vi "Untitled 1.vi"() -> ()   [LabVIEW 2017]
uses:
  <userlib>/_OpenG.lib/array/array.llb/Remove Duplicates from 1D Array (String)__ogtk.vi
  <userlib>/_OpenG.lib/array/array.llb/Index 1D Array Elements (String)__ogtk.vi
panel:
  out "Duplicates":string[](array[string])
  out "indices of removed elements":i32[](array[numeric])
  out "Array":string[](array[string])
  out "Error (out)":errorcluster
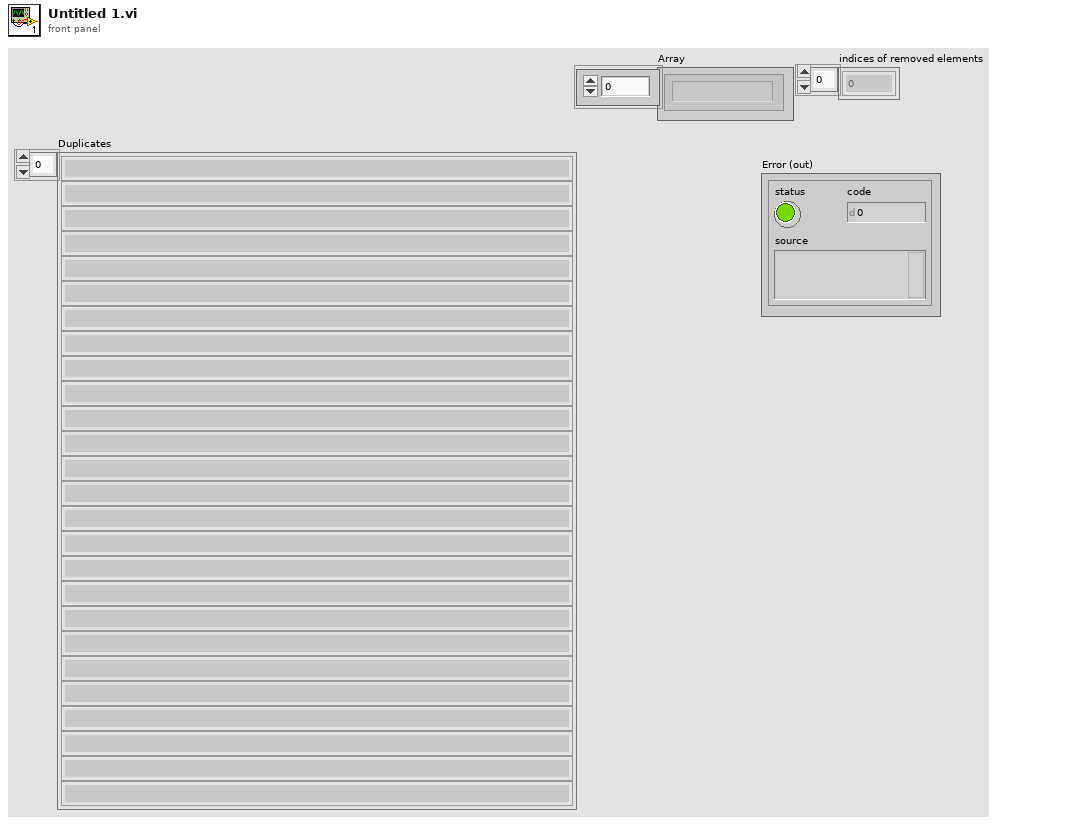
[diagram p1: front panel]
types:
  T1 = typedef "Database_Array.ctl" = cluster{"Core Number":i32, "Channel Number":i32, "Channel Name":string, "Channel Speed":i32, "Label Decimal":i32, "Label Name":string, "Min Rate (mS)":i32, "Max Rate (mS)":i32, "SDI":i32, "SSM":i32, "Create SDI":bool, "Create SSM":bool, "Create Parity":bool, "Parameter Name":string, "Start Bit":i32, "Number of Bits":i32, "Scale":string, "Offset":string, "Signed":bool, "Unit":string, "Encoding":T2, "Default Value":string}
  T2 = typedef "Encoding.ctl" = enum16{"BCD", "BNR", "Discrete"}
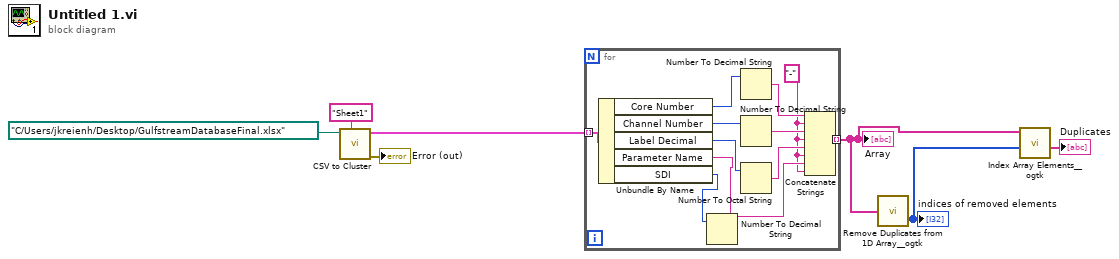
[diagram p0: block diagram]
diagram:
  n1 = call "CSV to Cluster.vi"("Excel._SheetName"="Sheet1", "file path (dialog if empty)"=path "C:/Users/jkreienh/Desktop/GulfstreamDatabaseFinal.xlsx") -> ("Error (out)"=→"Error (out)":errorcluster, "Parameter Array"=w4:T1[])  [unwired: 8 in]
  n2 = for {
    tunnel: w4 -> [w18] mode=indexing
    tunnel: [w11] -> w3 mode=indexing
    w9 = "-"
    n3 = Unbundle By Name(w18) -> ("Core Number"=w17:i32, "Channel Number"=w16:i32, "Label Decimal"=w15:i32, "Parameter Name"=w10:string, "SDI"=w8:i32)
    n4 = Number To Decimal String(number=w8) -> ()  [unwired: 1 in, 1 out]
    n5 = Number To Decimal String(number=w17) -> (decimal integer string=w14:string)  [unwired: 1 in]
    n6 = Number To Decimal String(number=w16) -> (decimal integer string=w13:string)  [unwired: 1 in]
    n7 = Number To Octal String(2:w15) -> (0:w12:string)  [unwired: 1 in]
    n8 = Concatenate Strings(w14, w9, w13, w9, w12, w9, w10, w9) -> (w11:string)
  }
  "Array" <- w3
  n9 = call-poly <userlib>:"Remove Duplicates from 1D Array__ogtk.vi"("Input Array"=w3) -> ("indices of removed elements"=w2:i32[])  [unwired: 1 out]
  "indices of removed elements" <- w2
  n10 = call-poly <userlib>:"Index Array Elements__ogtk.vi"("indices"=w2, "array"=w3) -> ("elements"=→"Duplicates":string[])  [unwired: 9 in]
